vi "Offline_Analysis_SVM_분석기.vi"(0 "LDA_matrix":path caption="LDA_matrix.txt", 1 "Target":path, 2 "Nontarget":path, 5 "Target_order.txt":path, 7 "mius_flash_order":path, 9 "Brain":path, 11 "svm_model_file":string, 12 "피험자이름":string="홍길동", 13 "Save_path":string) -> ()   [LabVIEW 2014]
uses:
  <vilib>/Utility/file.llb/Read From Spreadsheet File (DBL).vi
  <vilib>/Analysis/Matrix/Numeric/Conversions/Array To Matrix - RA2.vi
  <vilib>/Analysis/Matrix/Numeric/Conversions/Array To Matrix - RA.vi
  <vilib>/Utility/file.llb/Read From Spreadsheet File (I64).vi
  <vilib>/Utility/file.llb/Write To Spreadsheet File (DBL).vi
  <vilib>/Utility/file.llb/Write To Spreadsheet File (I64).vi
  <vilib>/Utility/file.llb/Write To Spreadsheet File (string).vi
  <vilib>/Analysis/Matrix/NI_Matrix.lvlib
panel:
  out "ACC":i16
  in  "Channel selection":bool[](array[boolean])=[TRUE, TRUE, TRUE, TRUE, TRUE, TRUE, TRUE, TRUE, TRUE, TRUE, TRUE]
  out "Target_order":i64[](array[numeric])
  out "Selected_Target":i32[](array[numeric])
  out "Accuracy":i16[](array[numeric])
  out "error out":errorcluster
  in  "Random_num":i32=6
  in  "Flash_Repeat":i32=20
  in  "Frame_Length":i32=10
  in  "Sampling_Rate":dbl=250.0
  # "ERP_Parameter안씀. LDA바로 집어넣으면 됨"
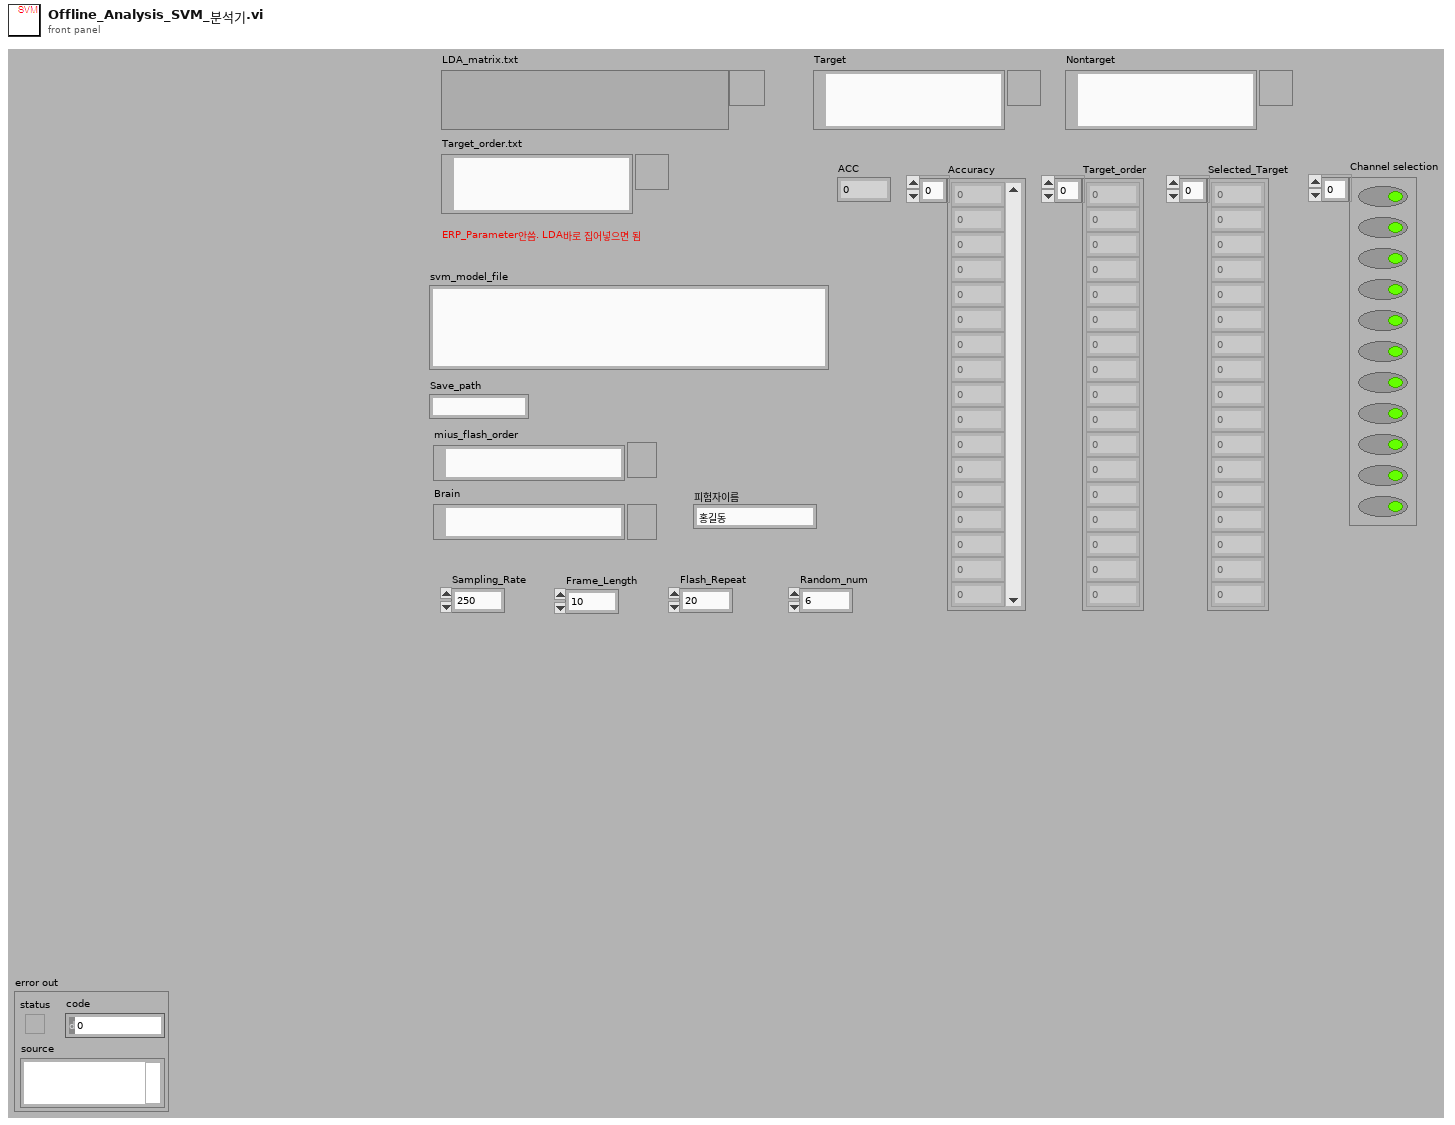
[diagram p1: front panel]
types:
  T1 = typedef "NI_Matrix.lvlib/RealMatrix.ctl" = dbl[][]
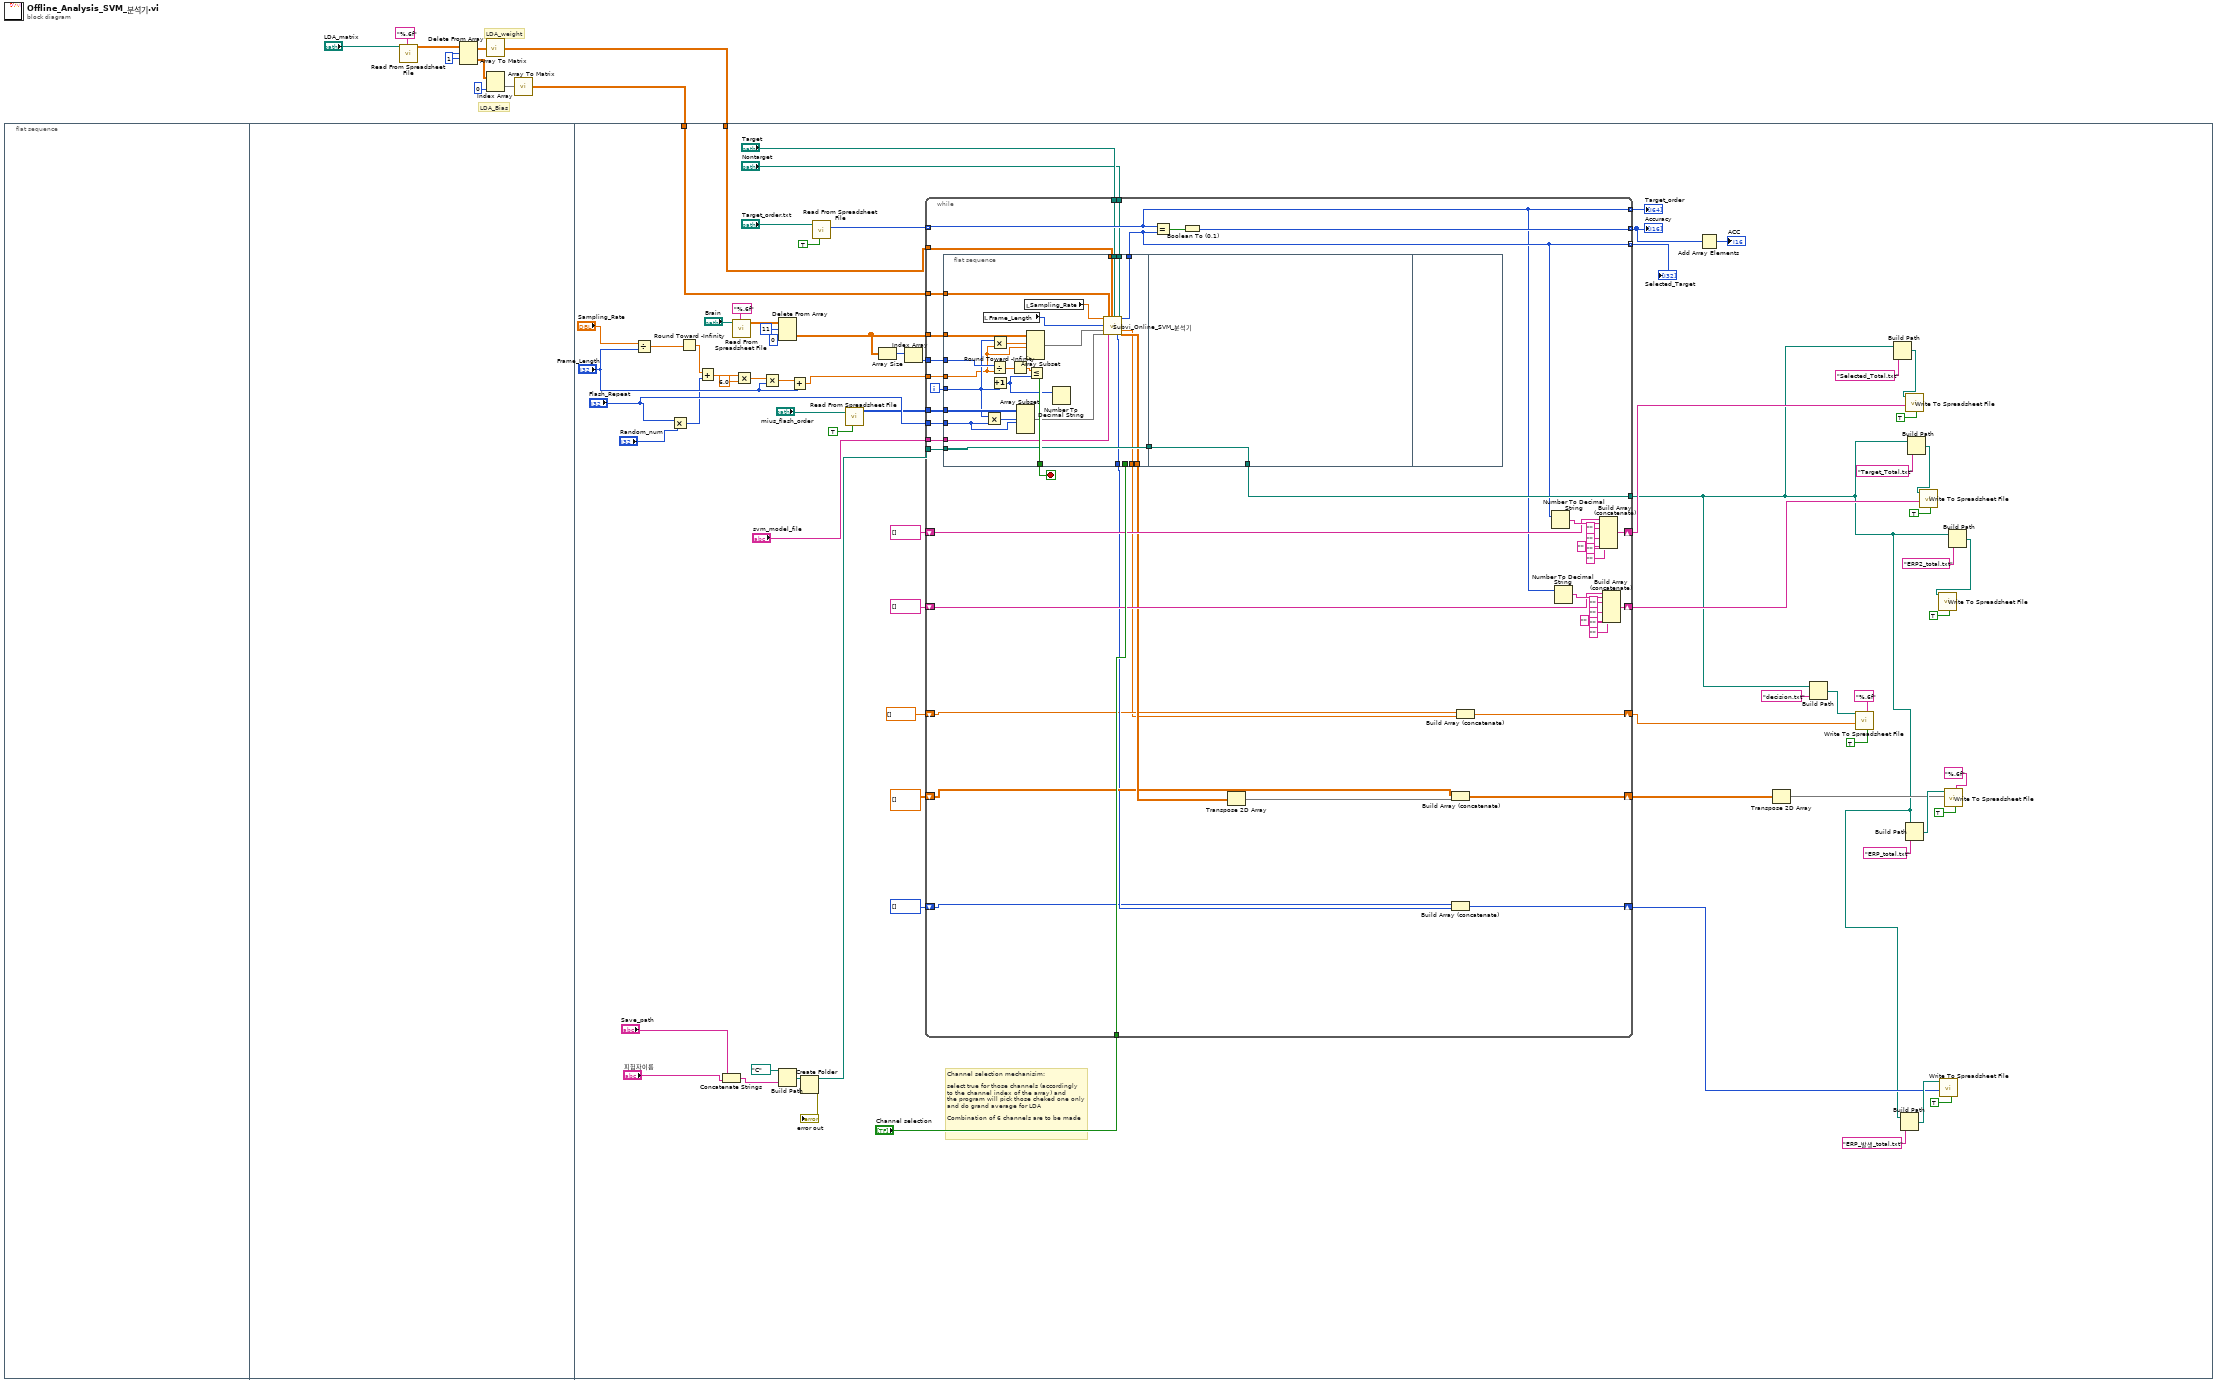
[diagram p0: block diagram]
diagram:
  w5 = 1 ("인덱스 (행)")
  # "LDA_Bias"
  # "LDA_weight"
  n1 = flat-sequence {
    tunnel: w2 -> [w25]
    tunnel: w1 -> [w24]
    frame #0 {
    }
    frame #1 {
    }
    frame #2 {
      # "Channel selection mechanisim:\n\nselect true for those channels (accordingly\nto the channel index of the array) and \nthe program will pick those cheked one only\nand do grand average for LDA\n\nCombination of 6 channels are to be made"
      n2 = Divide(x="Sampling_Rate", y="Frame_Length") -> (x/y=w69:dbl)
      n3 = Multiply(x="Flash_Repeat", y="Random_num") -> (x*y=w72:i32)
      n4 = Round Toward -Infinity(1:w69) -> (0:w71:dbl)
      n5 = Add(x=w71, y=w72) -> (x+y=w74:dbl)
      n6 = Concatenate Strings("Save_path", "피험자이름") -> (w15:string)
      n7 = call-poly <vilib>:"Read From Spreadsheet File.vi"("format (%.3f)"="%.6f", "file path (dialog if empty)"="Brain") -> ("all rows"=w63:dbl[][])  [unwired: 5 in, 4 out]
      n8 = Multiply(x=w74, y=6.0) -> (x*y=w76:dbl)
      n9 = Multiply(x=w76, y="Frame_Length") -> (x*y=w78:dbl)
      n10 = Build Path(base path=path "C:/" ("path"), name or relative path=w15) -> (appended path=w81:path)
      n11 = Delete From Array(array=w63, length=11 ("길이"), index (col)=0 ("비활성화된 인덱스 (열)")) -> (deleted portion=w23:dbl[][])  [unwired: 1 in, 1 out]
      n12 = Add(x=w78, y="Frame_Length") -> (x+y=w79:dbl)
      n13 = Create Folder(path (use dialog)=w81) -> (created path=w83:path, error out=→"error out":errorcluster)  [unwired: 2 in, 1 out]
      n14 = call-poly <vilib>:"Read From Spreadsheet File.vi"("transpose (no:F)"=TRUE, "file path (dialog if empty)"="Target_order.txt") -> ("first row"=w57:i64[])  [unwired: 5 in, 4 out]
      n15 = call-poly <vilib>:"Read From Spreadsheet File.vi"("transpose (no:F)"=TRUE, "file path (dialog if empty)"="mius_flash_order") -> ("all rows"=w65:i64[][])  [unwired: 5 in, 4 out]
      n16 = Array Size(array=w23) -> (size(s)=w66:i32[])
      n17 = Index Array(array=w66) -> (element=w67:i32)  [unwired: 1 in]
      n18 = while {
        tunnel: w24 -> [w131]
        tunnel: w25 -> [w130]
        tunnel: w23 -> [w128]
        tunnel: w65 -> [w127]
        tunnel: w67 -> [w129]
        tunnel: w79 -> [w125]
        tunnel: "Flash_Repeat" -> [w126]
        tunnel: w83 -> [w124]
        tunnel: w57 -> [w101] mode=indexing
        tunnel: [w121] -> w45 mode=indexing
        tunnel: [w101] -> w54 mode=indexing
        tunnel: [w102] -> w55 mode=indexing
        tunnel: "Channel selection" -> [w118]
        tunnel: [w117] -> w18
        shift-right: [w104] -> w39
        shift-left: string[] [] -> [w103]
        shift-right: [w100] -> w38
        shift-left: string[] [] -> [w99]
        shift-right: [w96] -> w33
        shift-left: dbl[][] [] -> [w95]
        shift-right: [w93] -> w26
        shift-left: i16[] [] -> [w92]
        shift-right: [w91] -> w17
        shift-left: dbl[] [] -> [w90]
        tunnel: "Target" -> [w88]
        tunnel: "Nontarget" -> [w87]
        tunnel: "svm_model_file" -> [w86]
        i -> [w120]
        stop <- w119 stop-if-true
        n19 = flat-sequence {
          tunnel: w131 -> [w157]
          tunnel: w130 -> [w135]
          tunnel: w129 -> [w156]
          tunnel: [w155] -> w119
          tunnel: w128 -> [w154]
          tunnel: w127 -> [w151]
          tunnel: w126 -> [w149]
          tunnel: w120 -> [w148]
          tunnel: w125 -> [w147]
          tunnel: w124 -> [w140]
          tunnel: [w140] -> w123
          tunnel: [w141] -> w102
          tunnel: w118 -> [_]
          tunnel: [w139] -> w98
          tunnel: [w138] -> w94
          tunnel: [w136] -> w89
          tunnel: w88 -> [w134]
          tunnel: w87 -> [w133]
          tunnel: w86 -> [w132]
          tunnel: w123 -> [w158]
          tunnel: [w158] -> w117
          frame #0 {
            n20 = local read "Frame_Length"() -> (w143:i32)
            n21 = Multiply(x=w148, y=w149) -> (x*y=w150:i32)
            n22 = Divide(x=w156, y=w147) -> (x/y=w146:dbl)
            n23 = Multiply(x=w148, y=w147) -> (x*y=w153:dbl)
            n24 = Increment(x=w148) -> (x+1=w142:i32)
            n25 = Round Toward -Infinity(1:w146) -> (0:w145:dbl)
            n26 = Array Subset(array=w151, index (row)=w150, length (row)=w149) -> (w137:i64[][])  [unwired: 2 in]
            n27 = local read "Sampling_Rate"() -> (w144:dbl)
            n28 = Array Subset(array=w154, index (row)=w153, length (row)=w147) -> (w152:dbl[][])  [unwired: 2 in]
            n29 = Less Or Equal?(x=w145, y=w142) -> (x <= y?=w155:bool)
            n30 = Number To Decimal String(number=w142) -> ()  [unwired: 1 in, 1 out]
            n31 = call "Subvi_Online_SVM_분석기.vi"("rate"=w144, "samples per channel"=w143, "Brain_data_source"=w152, "Target_Flash_Order"=w137, "Value 2"=w157, "svm_model_file"=w132, "Matrix 2"=w135, "Target"=w134, "Nontarget"=w133) -> ("EPR_발생_total"=w138:i16[], "output-0~8"=w141:i32, "decision"=w136:dbl[], "ERP_Parameters"=w139:dbl[][])  [unwired: 7 in]
          }
          frame #1 {
          }
          frame #2 {
          }
        }
        n32 = Equal?(x=w101, y=w102) -> (x = y?=w122:bool)
        n33 = Boolean To (0,1)(Boolean=w122) -> (0, 1=w121:i16)
        n34 = Transpose 2D Array(2D array=w98) -> (transposed array=w97:dbl[][])
        n35 = Build Array (concatenate)(w92, w94) -> (w93:i16[])
        n36 = Build Array (concatenate)(w95, w97) -> (w96:dbl[][])
        n37 = Build Array (concatenate)(w90, w89) -> (w91:dbl[])
        n38 = Number To Decimal String(number=w102) -> (decimal integer string=w110:string)  [unwired: 1 in]
        n39 = Number To Decimal String(number=w101) -> (decimal integer string=w116:string)  [unwired: 1 in]
        n40 = Build Array (concatenate)(w103, w110, "" ("element"), "" ("element"), "" ("element"), "" ("element"), "" ("element")) -> (w104:string[])
        n41 = Build Array (concatenate)(w99, w116, "" ("element"), "" ("element"), "" ("element"), "" ("element"), "" ("element")) -> (w100:string[])
      }
      "Accuracy" <- w45
      "Selected_Target" <- w55
      "Target_order" <- w54
      n42 = Add Array Elements(numeric array=w45) -> (sum=→"ACC":i16)
      n43 = Transpose 2D Array(2D array=w33) -> (transposed array=w31:dbl[][])
      n44 = Build Path(base path=w18, name or relative path="decision.txt") -> (appended path=w19:path)
      n45 = call-poly <vilib>:"Write To Spreadsheet File.vi"("transpose? (no:F)"=TRUE, "format (%.3f)"="%.6f", "1D data"=w17, "file path (dialog if empty)"=w19) -> ()  [unwired: 4 in, 1 out]
      n46 = Build Path(base path=w18, name or relative path="Selected_Total.txt") -> (appended path=w41:path)
      n47 = Build Path(base path=w18, name or relative path="ERP_발생_total.txt") -> (appended path=w28:path)
      n48 = call-poly <vilib>:"Write To Spreadsheet File.vi"("transpose? (no:F)"=TRUE, "1D data"=w39, "file path (dialog if empty)"=w41) -> ()  [unwired: 5 in, 1 out]
      n49 = Build Path(base path=w18, name or relative path="ERP_total.txt") -> (appended path=w34:path)
      n50 = Build Path(base path=w18, name or relative path="Target_Total.txt") -> (appended path=w47:path)
      n51 = call-poly <vilib>:"Write To Spreadsheet File.vi"("transpose? (no:F)"=TRUE, "1D data"=w38, "file path (dialog if empty)"=w47) -> ()  [unwired: 5 in, 1 out]
      n52 = call-poly <vilib>:"Write To Spreadsheet File.vi"("transpose? (no:F)"=TRUE, "1D data"=w26, "file path (dialog if empty)"=w28) -> ()  [unwired: 5 in, 1 out]
      n53 = call-poly <vilib>:"Write To Spreadsheet File.vi"("transpose? (no:F)"=TRUE, "format (%.3f)"="%.6f", "2D data"=w31, "file path (dialog if empty)"=w34) -> ()  [unwired: 4 in, 1 out]
      n54 = Build Path(base path=w18, name or relative path="ERP2_total.txt") -> (appended path=w49:path)
      n55 = call-poly <vilib>:"Write To Spreadsheet File.vi"("transpose? (no:F)"=TRUE, "file path (dialog if empty)"=w49) -> ()  [unwired: 6 in, 1 out]
    }
  }
  n56 = call-poly <vilib>:"Read From Spreadsheet File.vi"("format (%.3f)"="%.6f", "file path (dialog if empty)"="LDA_matrix") -> ("all rows"=w3:dbl[][])  [unwired: 5 in, 4 out]
  n57 = Delete From Array(array=w3, length=w5, index (row)=w5) -> (deleted portion=w8:dbl[][], array with subset deleted=w7:dbl[][])  [unwired: 1 in]
  n58 = call-poly <vilib>:"Array To Matrix.vi"("Real 2D Array"=w7) -> ("Real Matrix"=w2:T1)
  n59 = Index Array(array=w8, index (col)=0 ("인덱스")) -> (element=w6:dbl[])  [unwired: 1 in]
  n60 = call-poly <vilib>:"Array To Matrix.vi"("Real 1D Array"=w6) -> ("Real Matrix (Column Vector)"=w1:T1)
